vi "Measurement.Init.vi"(8 "error in (no error)":errorcluster, 10 "timeout (5000 ms)":i32=5000, 11 "Measurement in":refnum<class "Measurement.lvclass">) -> (0 "error out":errorcluster, 1 "Dependencies Results":bool[](array[boolean]), 2 "Result":bool, 3 "Measurement out":refnum<class "Measurement.lvclass">)   [LabVIEW 2017, in "Measurement.lvclass"]
uses:
  Measurement.lvclass
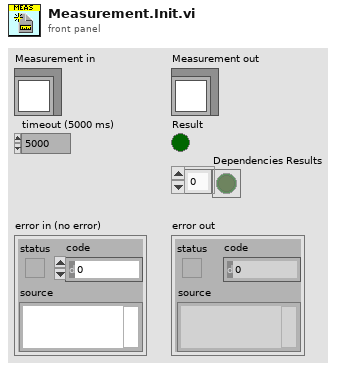
[diagram p1: front panel]
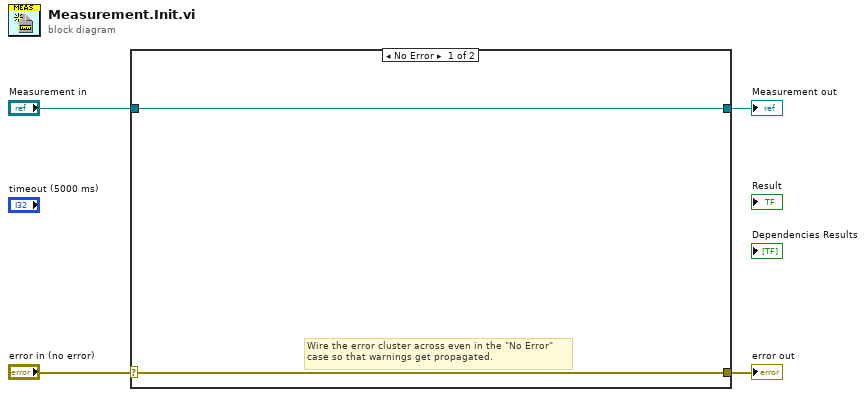
[diagram p0: block diagram]
diagram:
  n1 = case shown="No Error" "error in (no error)" {
    selector: "error in (no error)" -> [w5 w8]
    tunnel: [w5 w8] -> w3
    tunnel: [w6 w7] -> w1
    tunnel: "Measurement in" -> [w6 w7]
    frame No Error {
      # "Wire the error cluster across even in the \"No Error\"\ncase so that warnings get propagated."
    }
    frame Error {
    }
  }
  "error out" <- w3
  "Measurement out" <- w1
